vi "Logging Message Loop.vi"(8 "error in (no error)":errorcluster, 9 "Data Queue":refnum<queue>, 11 "Message Queues":T1) -> (0 "error out":errorcluster)   [LabVIEW 2014, in "PLS Logging.lvlib"]
doc: "The message loop subVI to handle messages pertaining to logging data."
uses:
  PLS Logging.lvlib
  support/Message Queue/All Message Queues.ctl
  support/Message Queue/Message Cluster.ctl
  Logging Configuration.ctl
  start info.ctl
  support/Message Queue/Enqueue Message (Single).vi
  <vilib>/Utility/error.llb/Error Cluster From Error Code.vi
  <vilib>/ErrorRing/Error Ring.xnode
  support/Message Queue/PLS Message Queue.lvlib
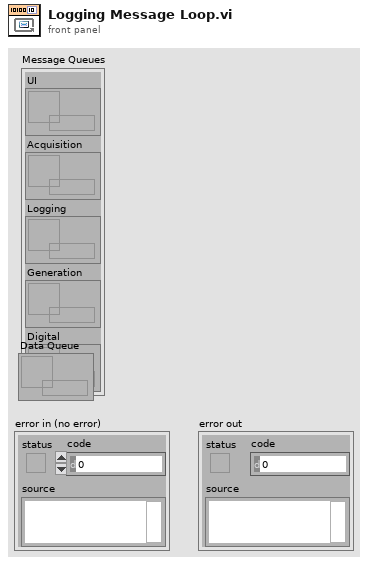
[diagram p1: front panel]
types:
  T1 = typedef "PLS Message Queue.lvlib/All Message Queues.ctl" = cluster{"UI":refnum<queue>, "Acquisition":refnum<queue>, "Logging":refnum<queue>, "Generation":refnum<queue>, "Digital":refnum<queue>}
  T2 = typedef "PLS Logging.lvlib/Logging Configuration.ctl" = cluster{"Log File Base Path":path, "L1":cluster{"ref":refnum<file>, "actif?":bool, "Fsave":i32}, "L2":cluster{"ref":refnum<file>, "actif?":bool, "Fsave":i32}, "L3":cluster{"ref":refnum<file>, "actif?":bool, "Fsave":i32}, "L4":cluster{"ref":refnum<file>, "actif?":bool, "Fsave":i32}}
  T3 = typedef "PLS Logging.lvlib/start info.ctl" = cluster{"path":path, "Fsave":i32, "#ligne":i32}
  T4 = enum16{"open", "replace", "create", "open or create", "replace or create", "replace or create with confirmation"}
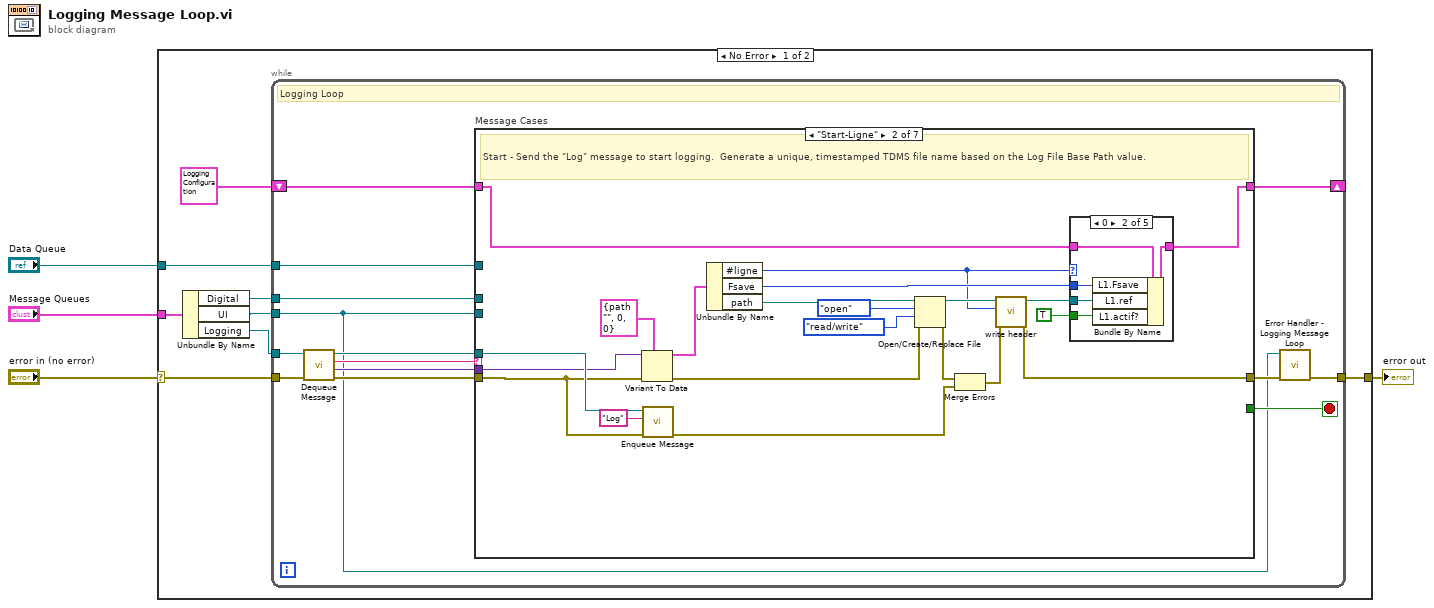
[diagram p0: block diagram]
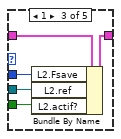
[diagram p4: hidden frame]
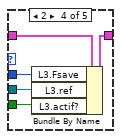
[diagram p5: hidden frame]
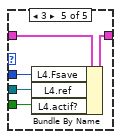
[diagram p6: hidden frame]
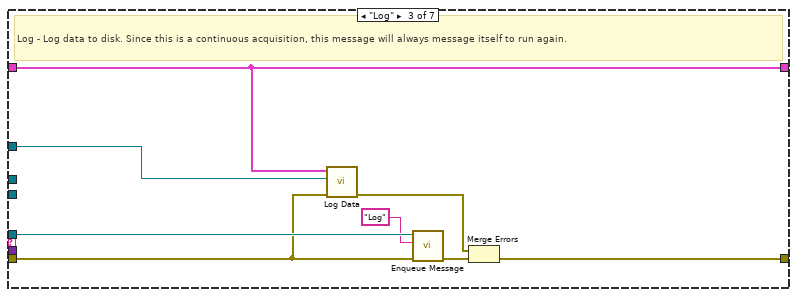
[diagram p7: hidden frame]
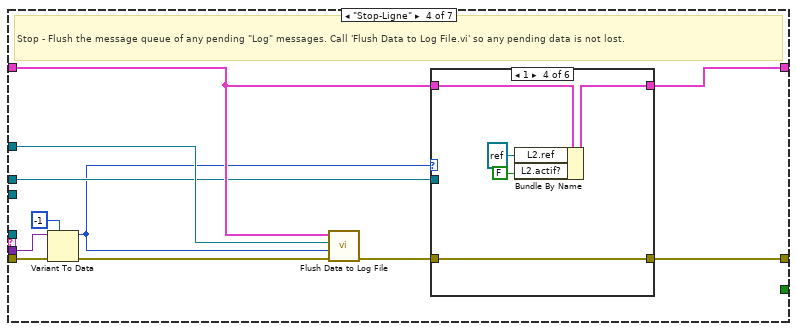
[diagram p8: hidden frame]
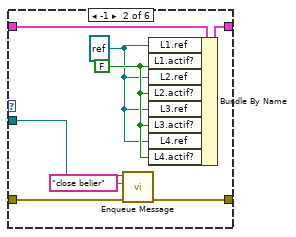
[diagram p10: hidden frame]
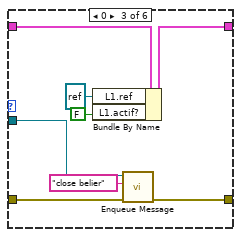
[diagram p11: hidden frame]
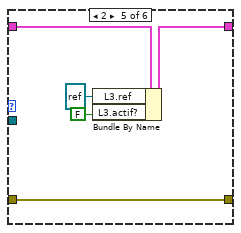
[diagram p12: hidden frame]
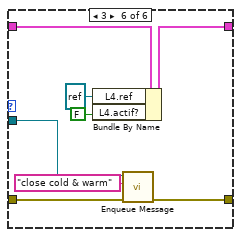
[diagram p13: hidden frame]
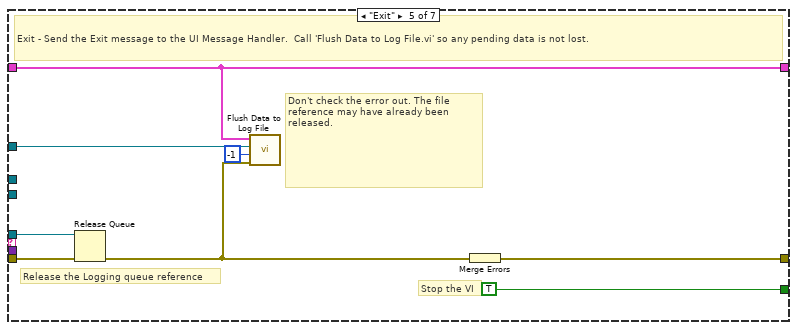
[diagram p14: hidden frame]
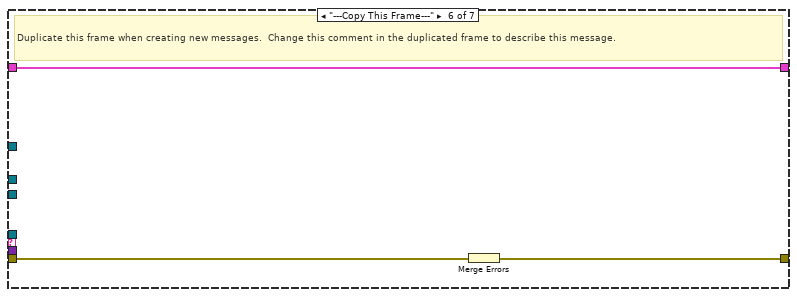
[diagram p15: hidden frame]
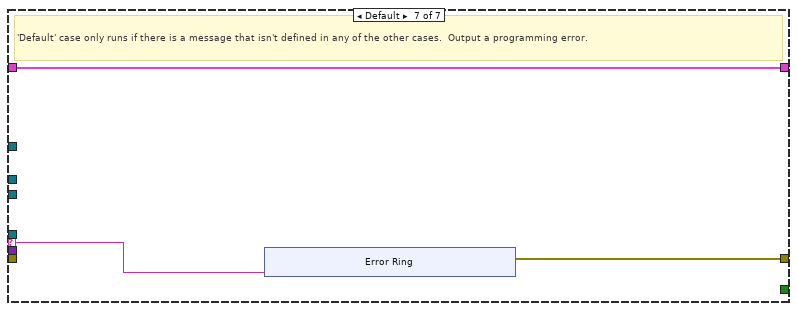
[diagram p16: hidden frame]
diagram:
  n1 = case shown="No Error" "error in (no error)" {
    selector: "error in (no error)" -> [w8 w147]
    tunnel: "Message Queues" -> [w12 _]
    tunnel: [w10 w147] -> w3
    tunnel: "Data Queue" -> [w7 _]
    frame No Error {
      n2 = Unbundle By Name(w12) -> ("Digital"=w5:refnum<queue>, "UI"=w6:refnum<queue>, "Logging"=w11:refnum<queue>)
      n3 = while {
        tunnel: w11 -> [w18]
        shift-right: [w25] -> _
        shift-left: T2 {"Log File Base Path"=path "", "L1"={"ref"=refnum, "actif?"=FALSE, "Fsave"=0}, "L2"={"ref"=refnum, "actif?"=FALSE, "Fsave"=0}, "L3"={"ref"=refnum, "actif?"=FALSE, "Fsave"=0}, "L4"={"ref"=refnum, "actif?"=FALSE, "Fsave"=0}} ("Logging Configuration") -> [w26]
        tunnel: w6 -> [w13]
        tunnel: w7 -> [w17]
        tunnel: w8 -> [w23]
        tunnel: [w16] -> w10
        tunnel: w5 -> [w14]
        stop <- w24 stop-if-true
        # "Logging Loop"
        n4 = call "Dequeue Message.vi"("error in (no error)"=w23, "Message Queue"=w18) -> ("error out"=w22:errorcluster, "Message Data"=w20:variant, "Message"=w21:string, "dup Message Queue"=w19:refnum<queue>)  [unwired: 6 in]
        n5 = case "Message Cases" shown="\"Start-Ligne\"" w21 {
          selector: w21 -> [_ _ _ _ _ _ w137]
          tunnel: w19 -> [_ w48 w77 _ w130 _ _]
          tunnel: w22 -> [w27 w47 w75 w86 w131 w136 _]
          tunnel: [w27 w49 w78 w81 w132 w134 w138] -> w15
          tunnel: w26 -> [w28 w46 w74 w88 w128 w135 w139]
          tunnel: [w28 w45 w74 w87 w128 w135 w139] -> w25
          tunnel: [_ _ _ _ TRUE _ _] -> w24
          tunnel: w20 -> [_ w44 _ w84 _ _ _]
          tunnel: w13 -> [_ _ _ _ _ _ _]
          tunnel: w17 -> [_ _ w76 w89 w127 _ _]
          tunnel: w14 -> [_ _ _ w82 _ _ _]
          frame "Initialize" {
            # "Initialize - gets called when first launched. Currently a no-op."
          }
          frame "Start-Ligne" {
            # "Start - Send the \"Log\" message to start logging.  Generate a unique, timestamped TDMS file name based on the Log File Base Path value."
            n6 = Variant To Data(error in=w47, type=T3 {"path"=path "", "Fsave"=0, "#ligne"=0} ("start info"), Variant=w44) -> (data=w34:T3, error out=w37:errorcluster)
            n7 = call-poly "Enqueue Message.vi"("error in (no error)"=w47, "Message"="Log", "Message Queue"=w48) -> ("error out"=w42:errorcluster)  [unwired: 7 in, 1 out]
            n8 = Unbundle By Name(w34) -> ("#ligne"=w29:i32, "Fsave"=w31:i32, "path"=w32:path)
            n9 = Open/Create/Replace File(file path (use dialog)=w32, error in=w37, operation (0:open)=T4."open", access (0:read/write)=enum16{"read/write", "read-only", "write-only"}."read/write") -> (refnum out=w40:refnum<file>, error out=w41:errorcluster)  [unwired: 2 in, 1 out]
            n10 = Merge Errors(w41, w42) -> (w35:errorcluster)
            n11 = call "write header.vi"("error in (no error)"=w35, "line #"=w29, "Byte Stream File in"=w40) -> ("error out"=w49:errorcluster, "Byte Stream File out"=w36:refnum<file>)  [unwired: 7 in]
            n12 = case shown="0" w29 {
              tunnel: [w50 w53 w58 w63 w68] -> w45
              tunnel: w46 -> [w50 w54 w59 w64 w69]
              tunnel: w36 -> [_ w55 w60 w65 w70]
              tunnel: w31 -> [_ w52 w57 w62 w67]
              tunnel: TRUE ("L3.actif?") -> [_ w51 w56 w61 w66]
              frame Default {
              }
              frame 0 {
                n13 = Bundle By Name(cluster=w54, "L1.Fsave"=w52, "L1.ref"=w55, "L1.actif?"=w51) -> (w53:T2)
              }
              frame 1 {
                n14 = Bundle By Name(cluster=w59, "L2.Fsave"=w57, "L2.ref"=w60, "L2.actif?"=w56) -> (w58:T2)
              }
              frame 2 {
                n15 = Bundle By Name(cluster=w64, "L3.Fsave"=w62, "L3.ref"=w65, "L3.actif?"=w61) -> (w63:T2)
              }
              frame 3 {
                n16 = Bundle By Name(cluster=w69, "L4.Fsave"=w67, "L4.ref"=w70, "L4.actif?"=w66) -> (w68:T2)
              }
            }
          }
          frame "Log" {
            # "Log - Log data to disk. Since this is a continuous acquisition, this message will always message itself to run again."
            n17 = call "Log Data.vi"("error in (no error)"=w75, "Data Queue"=w76, "Logging Configuration"=w74) -> ("error out"=w72:errorcluster)  [unwired: 8 in]
            n18 = call-poly "Enqueue Message.vi"("error in (no error)"=w75, "Message"="Log", "Message Queue"=w77) -> ("error out"=w73:errorcluster)  [unwired: 7 in, 1 out]
            n19 = Merge Errors(w72, w73) -> (w78:errorcluster)
          }
          frame "Stop-Ligne" {
            # "Stop - Flush the message queue of any pending \"Log\" messages. Call 'Flush Data to Log File.vi' so any pending data is not lost."
            n20 = Variant To Data(error in=w86, type=-1, Variant=w84) -> (data=w80:i32, error out=w85:errorcluster)
            n21 = call "Flush Data to Log File.vi"("error in (no error)"=w85, "id ligne"=w80, "Data Queue"=w89, "Logging Configuration"=w88) -> ("error out"=w79:errorcluster)  [unwired: 7 in]
            n22 = case shown="1" w80 {
              tunnel: w88 -> [w91 w99 w107 w112 w117 w125]
              tunnel: [w91 w98 w106 w111 w116 w124] -> w87
              tunnel: w82 -> [_ w97 w103 _ _ w118]
              tunnel: [w90 w94 w100 w108 w113 w120] -> w81
              tunnel: w79 -> [w90 w95 w101 w108 w113 w119]
              frame Default {
              }
              frame -1 {
                w93 = FALSE ("L1.actif?")
                w92 = refnum<file> refnum ("L1.ref")
                n23 = call-poly "Enqueue Message.vi"("error in (no error)"=w95, "Message"="close belier", "Message Queue"=w97) -> ("error out"=w94:errorcluster)  [unwired: 7 in, 1 out]
                n24 = Bundle By Name(cluster=w99, "L1.ref"=w92, "L1.actif?"=w93, "L2.ref"=w92, "L2.actif?"=w93, "L3.ref"=w92, "L3.actif?"=w93, "L4.ref"=w92, "L4.actif?"=w93) -> (w98:T2)
              }
              frame 0 {
                n25 = Bundle By Name(cluster=w107, "L1.ref"=refnum<file> refnum, "L1.actif?"=FALSE) -> (w106:T2)
                n26 = call-poly "Enqueue Message.vi"("error in (no error)"=w101, "Message"="close belier", "Message Queue"=w103) -> ("error out"=w100:errorcluster)  [unwired: 7 in, 1 out]
              }
              frame 1 {
                n27 = Bundle By Name(cluster=w112, "L2.ref"=refnum<file> refnum ("L1.ref"), "L2.actif?"=FALSE ("L1.actif?")) -> (w111:T2)
              }
              frame 2 {
                n28 = Bundle By Name(cluster=w117, "L3.ref"=refnum<file> refnum ("L1.ref"), "L3.actif?"=FALSE ("L1.actif?")) -> (w116:T2)
              }
              frame 3 {
                n29 = Bundle By Name(cluster=w125, "L4.ref"=refnum<file> refnum ("L1.ref"), "L4.actif?"=FALSE ("L1.actif?")) -> (w124:T2)
                n30 = call-poly "Enqueue Message.vi"("error in (no error)"=w119, "Message"="close cold & warm", "Message Queue"=w118) -> ("error out"=w120:errorcluster)  [unwired: 7 in, 1 out]
              }
            }
          }
          frame "Exit" {
            # "Don't check the error out. The file reference may have already been released."
            # "Release the Logging queue reference"
            # "Stop the VI"
            # "Exit - Send the Exit message to the UI Message Handler.  Call 'Flush Data to Log File.vi' so any pending data is not lost."
            n31 = Release Queue(queue=w130, error in (no error)=w131) -> (error out=w129:errorcluster)  [unwired: 1 in, 2 out]
            n32 = call "Flush Data to Log File.vi"("error in (no error)"=w129, "id ligne"=-1, "Data Queue"=w127, "Logging Configuration"=w128) -> ()  [unwired: 7 in, 1 out]
            n33 = Merge Errors(w129) -> (w132:errorcluster)
          }
          frame "---Copy This Frame---" {
            # "Duplicate this frame when creating new messages.  Change this comment in the duplicated frame to describe this message."
            n34 = Merge Errors(w136) -> (w134:errorcluster)
          }
          frame Default {
            # "'Default' case only runs if there is a message that isn't defined in any of the other cases.  Output a programming error."
            n35 = xnode "Error Ring"("parameter 0"=w137) -> ("error out"=w138:errorcluster)
          }
        }
        n36 = call "Error Handler - Logging Message Loop.vi"("error in (no error)"=w15, "Message Queue"=w13) -> ("dup error in"=w16:errorcluster)  [unwired: 8 in, 1 out]
      }
    }
    frame Error {
    }
  }
  "error out" <- w3
